vi "EXAMPLE_REGEXP.vi"() -> ()   [LabVIEW 2017]
uses:
  4f433c9a-a00c-49f1-9e84-35b769afccce.vi
  8cf9f43b-58a1-407a-9b53-072bd7cbe5d9.vi
  TagDB/_Support/DataAccess/_NameCacher.vi
  TagDB/_Support/DataAccess/_datatypeChecker.vi
  TagDB/_Support/Error/_Clear Errors.vi
  8cf9f43b-58a1-407a-9b53-072bd7cbe5d9.vi/29b2ea6d-6d7f-4e4a-ad31-a5cb760462c7.vi
  TagDB/API/TagDB-Status.vi
  TagDB/_Support/DataAccess/TagDB Ref to DVR.vi
  <vilib>/Utility/Data Type/Get Type Information.vi
  <vilib>/Utility/error.llb/Trim Whitespace.vi
  TagDB/_Support/Error/_[error50000]Invalid DB REF.vi
  TagDB/_Support/Change Detector/TagDB dbChanged.vi
  TagDB/_Support/Error/_[error50002]Invalid DataType.vi
  TagDB/TagDB(DEV).lvlib
panel:
  out "names Sorted":string[](array[string])
  out "value":i32[][](array[numeric])
  out "names":string[](array[string])
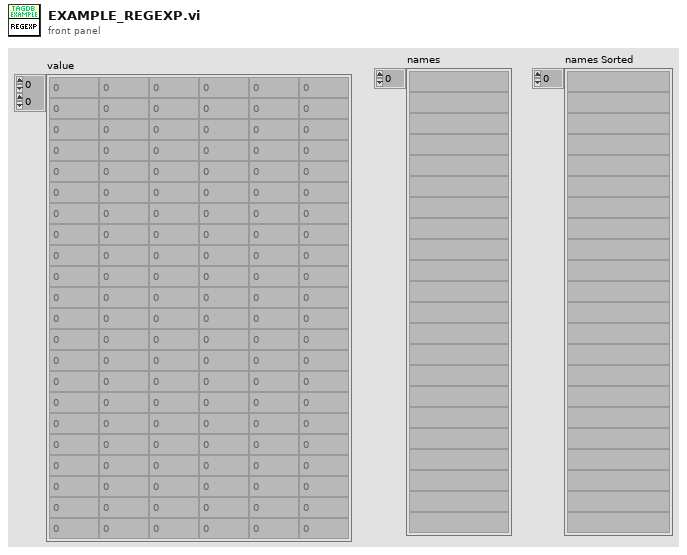
[diagram p1: front panel]
types:
  T1 = typedef "TagDB(DEV).lvlib/TagDB.ctl" = refnum<k1>
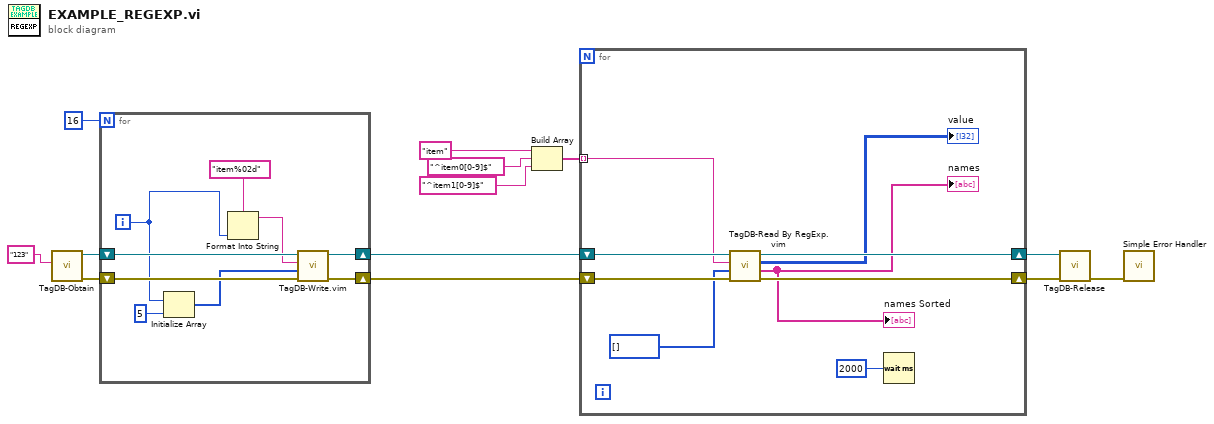
[diagram p0: block diagram]
diagram:
  n1 = call "TagDB-Obtain.vi"("name (unnamed)"="123") -> ("error out"=w9:errorcluster, "TagDB"=w10:T1)  [unwired: 4 in, 1 out]
  n2 = for {
    N: 16 -> [_]
    shift-right: [w20] -> w12
    shift-left: w10 -> [w22]
    shift-right: [w19] -> w11
    shift-left: w9 -> [w21]
    i -> [w15]
    n3 = Initialize Array(w15, 5 ("dimension size")) -> (w16:i32[])
    n4 = Format Into String(format string="item%02d" ("String"), w15) -> (resulting string=w17:string)  [unwired: 2 in, 1 out]
    n5 = call "TagDB-Write.vim"("error in (no error)"=w21, "Value"=w16, "name"=w17, "TagDB"=w22) -> ("error out"=w19:errorcluster, "TagDB(dup)"=w20:T1)  [unwired: 5 in, 1 out]
  }
  n6 = Build Array("item", "^item0[0-9]$", "^item1[0-9]$") -> (w3:string[])
  n7 = for {
    shift-right: [w31] -> w1
    shift-left: w12 -> [w29]
    shift-right: [w30] -> w13
    shift-left: w11 -> [w28]
    tunnel: w3 -> [w23] mode=indexing
    n8 = call "TagDB-Read By RegExp.vim"("error in (no error)"=w28, "Type"=i32[] [], "RegExp"=w23, "DB Ref"=w29) -> ("error out"=w30:errorcluster, "names"=→"names" →"names Sorted":string[], "value"=→"value":i32[][], "DB Ref(dup)"=w31:T1)  [unwired: 4 in]
    n9 = Wait (ms)(milliseconds to wait=u32 2000) -> ()  [unwired: 1 out]
  }
  n10 = call "TagDB-Release.vi"("error in (no error)"=w13, "TagDB"=w1) -> ("error out"=w2:errorcluster)  [unwired: 9 in]
  n11 = call <vilib>:"Simple Error Handler.vi"("error in (no error)"=w2) -> ()  [unwired: 4 in, 5 out]
